vi "Main.vi"   [LabVIEW 2017]
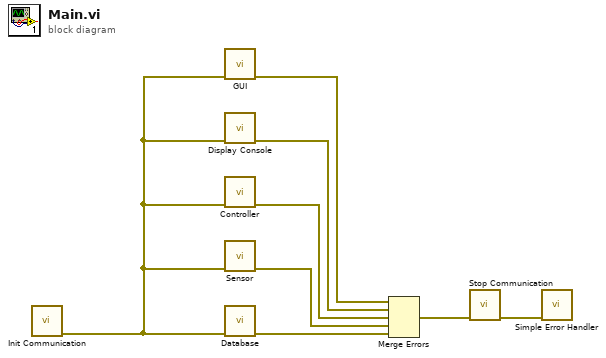
[diagram p0: block diagram]
diagram:
  n1 = call "Init Communication.vi"() -> ("error out"=w8:errorcluster)  [unwired: 11 in]
  n2 = call "GUI.vi"("error in (no error)"=w8) -> ("error out"=w3:errorcluster)  [unwired: 10 in]
  n3 = call "Display Console.vi"("error in (no error)"=w8) -> ("error out"=w4:errorcluster)  [unwired: 10 in]
  n4 = call "Controller.vi"("error in (no error)"=w8) -> ("error out"=w5:errorcluster)  [unwired: 10 in]
  n5 = call "Sensor.vi"("error in (no error)"=w8) -> ("error out"=w6:errorcluster)  [unwired: 10 in]
  n6 = call "Database.vi"("error in (no error)"=w8) -> ("error out"=w7:errorcluster)  [unwired: 10 in]
  n7 = Merge Errors(w3, w4, w5, w6, w7) -> (w2:errorcluster)
  n8 = call "Stop Communication.vi"("error in (no error)"=w2) -> ("error out"=w1:errorcluster)  [unwired: 10 in]
  n9 = call <vilib>:"Simple Error Handler.vi"("error in (no error)"=w1) -> ()  [unwired: 4 in, 5 out]
